vi "[FPGA] Create Local FPGA Memory.vi"() -> (3 "FPGA Memory":T1={"Analog Inputs"="Analog Inputs", "Conditioned AI"="Conditioned AI", "Analog Outputs (FXP(20,5))"="Analog Outputs (FXP(20,5))", "Analog Outputs (U16)"="Analog Outputs (U16)", "Digital Inputs"="Digital Inputs", "Digital Outputs"="Digital Outputs", "eHS Outputs - Lane 1"="eHS Outputs - Lane 1", "eHS Outputs - Lane 2"="eHS Outputs - Lane 2", "eHS Outputs - Lane 3"="eHS Outputs - Lane 3", "SWG Signals"="SWG Outputs", "PWM Signals"="PWM Outputs", "SPWM Signals"="SPWM Outputs"})   [LabVIEW 2017]
uses:
  Controls/[FPGA] Local FPGA Memory.ctl
  <vilib>/rvi/DataTransferAndStorage/Container/Common/niFpgaContainerGetUniqueNameForEmu.vi
  <vilib>/rvi/DataTransferAndStorage/Container/Common/niFpgaContainerSetEmuInfo.vi
  <vilib>/rvi/eio/common/nirviEmuReportErrorAndStop.vi
  <vilib>/rvi/LocalResourceManager/LocalResourceManager.xnode
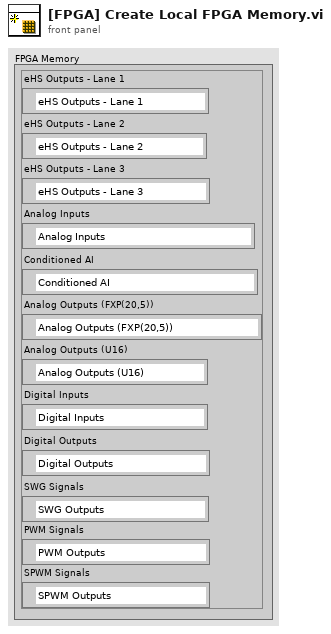
[diagram p1: front panel]
types:
  T1 = typedef "[FPGA] Local FPGA Memory.ctl" = cluster{"Analog Inputs":refnum<k21>, "Conditioned AI":refnum<k21>, "Analog Outputs (FXP(20,5))":refnum<k21>, "Analog Outputs (U16)":refnum<k21>, "Digital Inputs":refnum<k21>, "Digital Outputs":refnum<k21>, "eHS Outputs - Lane 1":refnum<k21>, "eHS Outputs - Lane 2":refnum<k21>, "eHS Outputs - Lane 3":refnum<k21>, "SWG Signals":refnum<k21>, "PWM Signals":refnum<k21>, "SPWM Signals":refnum<k21>}
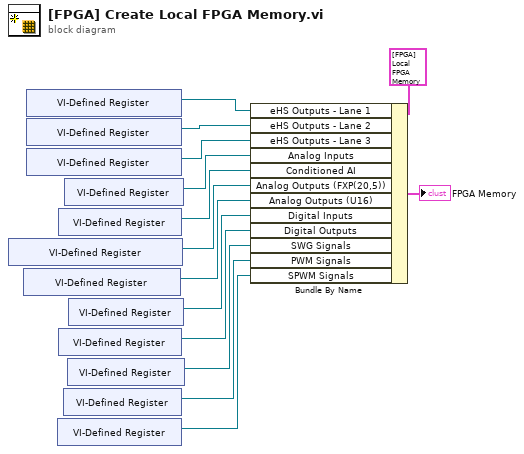
[diagram p0: block diagram]
diagram:
  n1 = xnode "VI-Defined Register"() -> ("Register Out"=w7:refnum<k21>)
  n2 = xnode "VI-Defined Register"() -> ("Register Out"=w6:refnum<k21>)
  n3 = xnode "VI-Defined Register"() -> ("Register Out"=w12:refnum<k21>)
  n4 = xnode "VI-Defined Register"() -> ("Register Out"=w11:refnum<k21>)
  n5 = xnode "VI-Defined Register"() -> ("Register Out"=w10:refnum<k21>)
  n6 = xnode "VI-Defined Register"() -> ("Register Out"=w1:refnum<k21>)
  n7 = xnode "VI-Defined Register"() -> ("Register Out"=w8:refnum<k21>)
  n8 = xnode "VI-Defined Register"() -> ("Register Out"=w4:refnum<k21>)
  n9 = xnode "VI-Defined Register"() -> ("Register Out"=w2:refnum<k21>)
  n10 = xnode "VI-Defined Register"() -> ("Register Out"=w9:refnum<k21>)
  n11 = xnode "VI-Defined Register"() -> ("Register Out"=w3:refnum<k21>)
  n12 = xnode "VI-Defined Register"() -> ("Register Out"=w5:refnum<k21>)
  n13 = Bundle By Name(cluster=T1 {"Analog Inputs"="", "Conditioned AI"="", "Analog Outputs (FXP(20,5))"="", "Analog Outputs (U16)"="", "Digital Inputs"="", "Digital Outputs"="", "eHS Outputs - Lane 1"="", "eHS Outputs - Lane 2"="", "eHS Outputs - Lane 3"="", "SWG Signals"="SWG Outputs", "PWM Signals"="PWM Outputs", "SPWM Signals"="SPWM Outputs"} ("Local FPGA Memory"), "eHS Outputs - Lane 1"=w12, "eHS Outputs - Lane 2"=w11, "eHS Outputs - Lane 3"=w10, "Analog Inputs"=w9, "Conditioned AI"=w8, "Analog Outputs (FXP(20,5))"=w7, "Analog Outputs (U16)"=w6, "Digital Inputs"=w5, "Digital Outputs"=w4, "SWG Signals"=w3, "PWM Signals"=w2, "SPWM Signals"=w1) -> (→"FPGA Memory":T1)
